vi "DWF Dig Read.vi"(0 "Instrument Handle In":u32, 5 "Lines":string, 11 "Error In":errorcluster caption="Error In (no error)") -> (4 "Instrument Handle Out":u32, 8 "Data":bool[](array[boolean]), 15 "Error Out":errorcluster)   [LabVIEW 2015, in "DigilentWF.lvlib"]
doc: "Reads the current state of the specified lines."
uses:
  <vilib>/DigilentWF/DigilentWF.lvlib
  dwf.dll
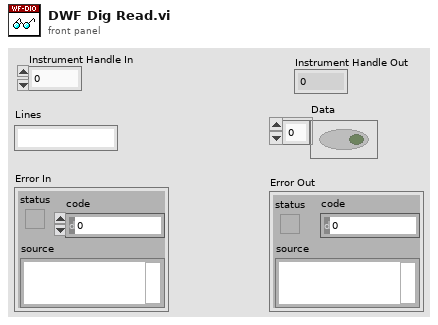
[diagram p1: front panel]
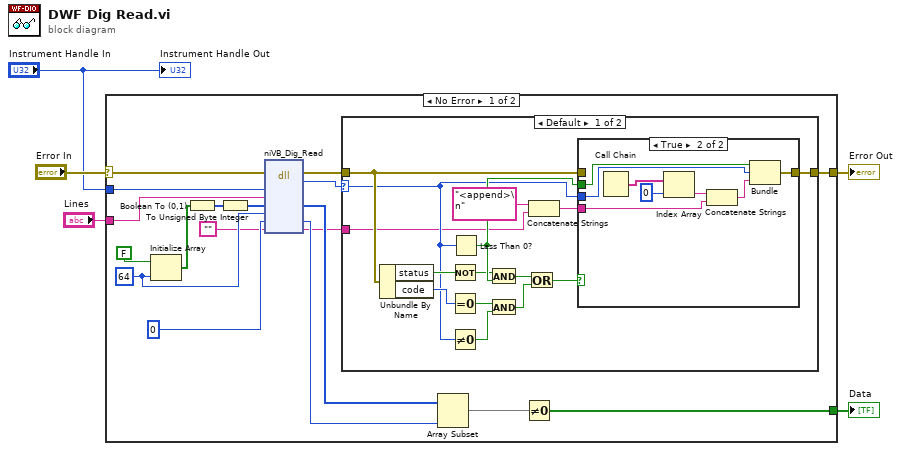
[diagram p0: block diagram]
diagram:
  n1 = case "outter_case" shown="No Error" "Error In" {
    selector: "Error In" -> [w21 w49]
    tunnel: [w23 w49] -> w4
    tunnel: "Lines" -> [w18 _]
    tunnel: [w22 _] -> w2
    tunnel: "Instrument Handle In" -> [w6 _]
    frame No Error {
      w12 = 64 ("dimension size")
      n2 = Initialize Array(FALSE, w12) -> (w13:bool[])
      n3 = Boolean To (0,1)(Boolean=w13) -> (0, 1=w10:i16[])
      n4 = To Unsigned Byte Integer(number=w10) -> (unsigned 8bit integer=w9:u8[])
      n5 = dll-call lib="dwf.*" fn="niVB_Dig_Read"(error in=w21, "instrumentHandle"=w6, "lines"=w18, "data"=w9, "dataSize"=w12, "dataSizeOut"=0, "szError"="") -> (error out=w20:errorcluster, "return type"=w19:i32, "data"=w17:u8[], "dataSizeOut"=w15:i32, "szError"=w7:string)  [unwired: 5 in, 1 out]
      n6 = case "inner_case" shown="Default" w19 {
        selector: w19 -> [w28 _]
        tunnel: w20 -> [w29 w48]
        tunnel: [w25 w48] -> w23
        tunnel: w7 -> [w24 _]
        frame Default {
          n7 = Unbundle By Name(w29) -> ("status"=w33:bool, "code"=w37:i32)
          n8 = Not(x=w33) -> (.not. x?=w36:bool)
          n9 = Equal To 0?(x=w37) -> (x = 0?=w32:bool)
          n10 = Not Equal To 0?(x=w28) -> (x != 0?=w35:bool)
          n11 = Less Than 0?(x=w28) -> (x < 0?=w38:bool)
          n12 = And(x=w36, y=w38) -> (x .and. y?=w34:bool)
          n13 = And(x=w32, y=w35) -> (x .and. y?=w31:bool)
          n14 = Or(x=w34, y=w31) -> (x .or. y?=w30:bool)
          n15 = Concatenate Strings("<append>\n" ("string"), w24) -> (w27:string)
          n16 = case shown="True" w30 {
            tunnel: [w39 w46] -> w25
            tunnel: w28 -> [_ w45]
            tunnel: w38 -> [_ w44]
            tunnel: w29 -> [w39 _]
            tunnel: w27 -> [_ w40]
            frame False {
            }
            frame True {
              n17 = Call Chain() -> (call chain=w43:string[])
              n18 = Index Array(array=w43, index=0) -> (element=w42:string)
              n19 = Concatenate Strings(w42, w40) -> (w47:string)
              n20 = Bundle(w44, "return type"=w45, w47) -> (w46:cluster{bool, "return type":i32, string})  [unwired: 1 out]
            }
          }
        }
        frame 0 {
        }
      }
      n21 = Array Subset(array=w17, length=w15) -> (w16:u8[])  [unwired: 1 in]
      n22 = Not Equal To 0?(x=w16) -> (x != 0?=w22:bool[])
    }
    frame Error {
    }
  }
  "Error Out" <- w4
  "Data" <- w2
  "Instrument Handle Out" <- "Instrument Handle In"
